vi "Add PID Controller.vi"(8 "error in (no error)":errorcluster, 11 "Node Ptr":u64 format="%.0x") -> (0 "error out":errorcluster, 2 "Controller PID Parameters Ref":T1 format="%.0x", 3 "Controller Ref Out":T1 format="%.0x")   [LabVIEW 2019, in "Control Addon System Explorer.lvlib"]
uses:
  Control Addon System Explorer.lvlib
  <vilib>/NI VeriStand/Custom Device API/Custom Device Item Ref.ctl
  <vilib>/NI VeriStand/Custom Device API/Custom Device Channel.ctl
  <vilib>/NI VeriStand/Custom Device API/Custom Device Channel Type.ctl
  Types/Action.ctl
  Addon Shared/Types/Controller Settings.ctl
  Addon Shared/SubVIs/Constants.vi
  <vilib>/NI VeriStand/Custom Device API/NI VeriStand - Get Item Property.vi
  <vilib>/NI VeriStand/Custom Device API/Get Item Property (Double).vi
  <vilib>/NI VeriStand/Custom Device API/Get Item Property (Boolean).vi
  <vilib>/NI VeriStand/Custom Device API/NI VeriStand - Set Item Property.vi
  <vilib>/NI VeriStand/Custom Device API/Set Item Property (Double).vi
  <vilib>/NI VeriStand/Custom Device API/Set Item Property (Boolean).vi
  <vilib>/NI VeriStand/Custom Device API/Custom Device API.lvlib
  Addon Shared/Control Addon Shared.lvlib
  Addon Shared/Types/PID Parameters.ctl
panel:
  in  "Tag":string
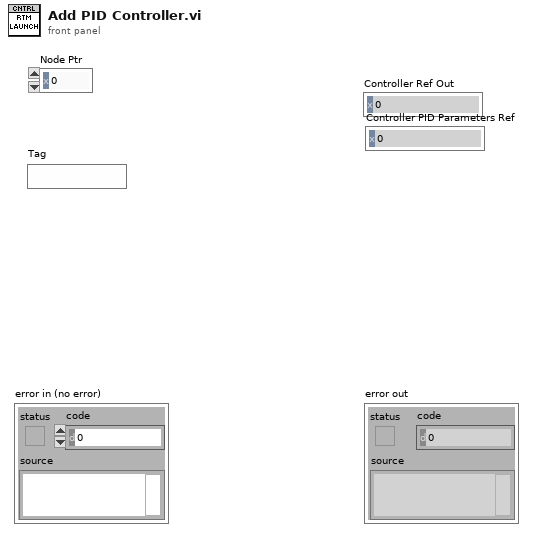
[diagram p1: front panel]
types:
  T1 = typedef "Custom Device API.lvlib/Custom Device Item Ref.ctl" = u64
  T2 = typedef "Control Addon Shared.lvlib/PID Parameters.ctl" = cluster{"Enable Live Updates":bool, "Enable Gain Scheduling":bool, "PID Parameters":dbl[][]}
  T3 = typedef "Control Addon System Explorer.lvlib/Action.ctl" = enum16{"Get", "Set"}
  T4 = typedef "Control Addon Shared.lvlib/Controller Settings.ctl" = cluster{"Output Max":dbl, "Output Min":dbl, "Setpoint Max":dbl, "Setpoint Min":dbl, "Use External Setpoint":bool, "Output Rate Limiter":dbl}
  T5 = typedef "Custom Device API.lvlib/Custom Device Channel.ctl" = cluster{"Type":T6, "Units":string, "Default Value":dbl, "Faultable":bool, "Scalable":bool}
  T6 = typedef "Custom Device API.lvlib/Custom Device Channel Type.ctl" = enum16{"Input", "Output"}
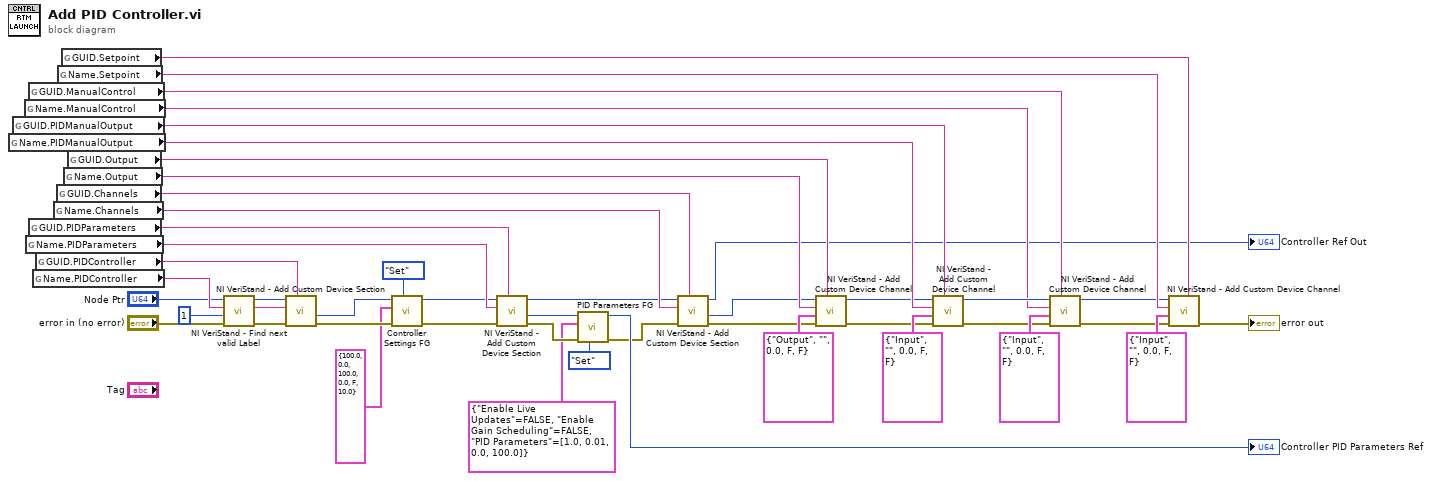
[diagram p0: block diagram]
diagram:
  n1 = global read "Constants.vi" "Name.PIDManualOutput"() -> (w24:string)
  n2 = global read "Constants.vi" "GUID.PIDManualOutput"() -> (w20:string)
  n3 = global read "Constants.vi" "Name.ManualControl"() -> (w23:string)
  n4 = global read "Constants.vi" "Name.PIDParameters"() -> (w44:string)
  n5 = global read "Constants.vi" "GUID.ManualControl"() -> (w22:string)
  n6 = global read "Constants.vi" "GUID.PIDParameters"() -> (w43:string)
  n7 = global read "Constants.vi" "Name.PIDController"() -> (w40:string)
  n8 = global read "Constants.vi" "GUID.PIDController"() -> (w47:string)
  n9 = global read "Constants.vi" "Name.Channels"() -> (w31:string)
  n10 = global read "Constants.vi" "GUID.Channels"() -> (w32:string)
  n11 = global read "Constants.vi" "Name.Setpoint"() -> (w41:string)
  n12 = global read "Constants.vi" "GUID.Setpoint"() -> (w19:string)
  n13 = global read "Constants.vi" "Name.Output"() -> (w42:string)
  n14 = global read "Constants.vi" "GUID.Output"() -> (w21:string)
  n15 = call <vilib>:"NI VeriStand - Find next valid Label.vi"("error in (no error)"="error in (no error)", "Start Value (1)"=1, "Label"=w40, "Item Ref in"="Node Ptr") -> ("error out"=w35:errorcluster, "Label out"=w39:string, "Item Ref out"=w37:T1)  [unwired: 3 in, 2 out]
  n16 = call <vilib>:"NI VeriStand - Add Custom Device Section.vi"("GUID (Default Section)"=w47, "error in (no error)"=w35, "Section Name"=w39, "Parent Ref in"=w37) -> ("error out"=w11:errorcluster, "Section Ptr"=w9:T1)  [unwired: 4 in, 2 out]
  n17 = call "Controller Settings FG.vi"("Action"=Action."Set", "error in (no error)"=w11, "Controller Settings"=T4 {"Output Max"=100.0, "Output Min"=0.0, "Setpoint Max"=100.0, "Setpoint Min"=0.0, "Use External Setpoint"=FALSE, "Output Rate Limiter"=10.0}, "Node Ptr"=w9) -> ("error out"=w10:errorcluster, "Item Ref out"=w8:T1)  [unwired: 5 in, 1 out]
  n18 = call <vilib>:"NI VeriStand - Add Custom Device Section.vi"("GUID (Default Section)"=w43, "error in (no error)"=w10, "Section Name"=w44, "Parent Ref in"=w8) -> ("error out"=w3:errorcluster, "Section Ptr"=w5:T1, "Parent Ref out"=w29:T1)  [unwired: 4 in, 1 out]
  n19 = call "PID Parameters FG.vi"("Action"=Action."Set", "error in (no error)"=w3, "Parameters"=T2 {"Enable Live Updates"=FALSE, "Enable Gain Scheduling"=FALSE, "PID Parameters"=[[1.0, 0.01, 0.0, 100.0]]}, "Node Ptr"=w5) -> ("error out"=w2:errorcluster, "Item Ref out"=→"Controller PID Parameters Ref":T1)  [unwired: 5 in, 1 out]
  n20 = call <vilib>:"NI VeriStand - Add Custom Device Section.vi"("GUID (Default Section)"=w32, "error in (no error)"=w2, "Section Name"=w31, "Parent Ref in"=w29) -> ("error out"=w34:errorcluster, "Section Ptr"=w33:T1, "Parent Ref out"=→"Controller Ref Out":T1)  [unwired: 4 in, 1 out]
  n21 = call <vilib>:"NI VeriStand - Add Custom Device Channel.vi"("GUID (Default Channel)"=w21, "error in (no error)"=w34, "Channel"=T5 {"Type"=enum."Output", "Units"="", "Default Value"=0.0, "Faultable"=FALSE, "Scalable"=FALSE}, "Channel Name"=w42, "Parent Ref in"=w33) -> ("error out"=w17:errorcluster, "Parent Ref out"=w18:T1)  [unwired: 3 in, 2 out]
  n22 = call <vilib>:"NI VeriStand - Add Custom Device Channel.vi"("GUID (Default Channel)"=w20, "error in (no error)"=w17, "Channel"=T5 {"Type"=enum."Input", "Units"="", "Default Value"=0.0, "Faultable"=FALSE, "Scalable"=FALSE}, "Channel Name"=w24, "Parent Ref in"=w18) -> ("error out"=w26:errorcluster, "Parent Ref out"=w25:T1)  [unwired: 3 in, 2 out]
  n23 = call <vilib>:"NI VeriStand - Add Custom Device Channel.vi"("GUID (Default Channel)"=w22, "error in (no error)"=w26, "Channel"=T5 {"Type"=enum."Input", "Units"="", "Default Value"=0.0, "Faultable"=FALSE, "Scalable"=FALSE}, "Channel Name"=w23, "Parent Ref in"=w25) -> ("error out"=w15:errorcluster, "Parent Ref out"=w14:T1)  [unwired: 3 in, 2 out]
  n24 = call <vilib>:"NI VeriStand - Add Custom Device Channel.vi"("GUID (Default Channel)"=w19, "error in (no error)"=w15, "Channel"=T5 {"Type"=enum."Input", "Units"="", "Default Value"=0.0, "Faultable"=FALSE, "Scalable"=FALSE}, "Channel Name"=w41, "Parent Ref in"=w14) -> ("error out"=→"error out":errorcluster)  [unwired: 3 in, 3 out]
